vi "Read Cal Files by Name.vi"(8 "Error In (no error)":errorcluster, 9 "Channel (1)":i32=1, 11 "VISA Resource Name":refnum<visa-resource-name>) -> (0 "error out":errorcluster, 1 "Cal Files by name":string[](array[string]), 3 "VISA Resource Out":refnum<visa-resource-name>)   [LabVIEW 2019, in "N5222A PNA.lvclass"]
uses:
  N5222A PNA.lvclass
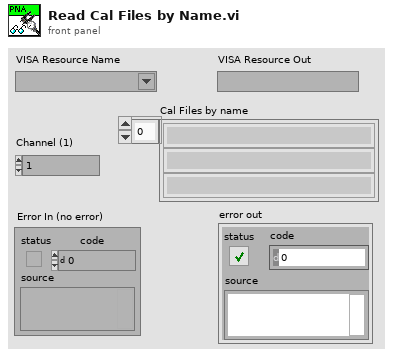
[diagram p1: front panel]
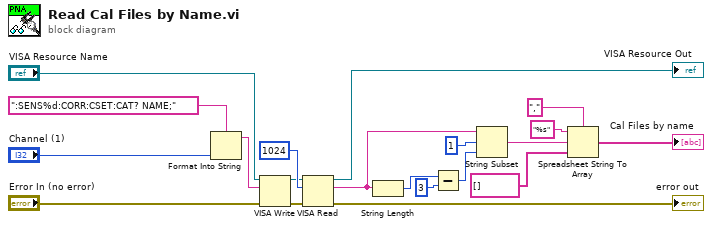
[diagram p0: block diagram]
diagram:
  n1 = Format Into String(format string=":SENS%d:CORR:CSET:CAT? NAME;", "Channel (1)") -> (resulting string=w20:string)  [unwired: 2 in, 1 out]
  n2 = VISA Write(VISA resource name="VISA Resource Name", write buffer=w20, error in (no error)="Error In (no error)") -> (VISA resource name out=w8:refnum<visa-resource-name>, error out=w9:errorcluster)  [unwired: 1 out]
  n3 = VISA Read(VISA resource name=w8, byte count=u32 1024 ("byte count (0)"), error in (no error)=w9) -> (VISA resource name out=→"VISA Resource Out":refnum<visa-resource-name>, read buffer=w18:string, error out=→"error out":errorcluster)  [unwired: 1 out]
  n4 = String Length(string=w18) -> (length=w15:i32)
  n5 = Subtract(x=w15, y=3) -> (x-y=w17:i32)
  n6 = String Subset(string=w18, offset (0)=1, length (rest)=w17) -> (substring=w19:string)
  n7 = Spreadsheet String To Array(delimiter (Tab)=",", format string="%s", spreadsheet string=w19, array type (2D Dbl)=string[] []) -> (array=→"Cal Files by name":string[])
